vi "Taiko_Init.vi"(8 "error in (no error)":errorcluster, 9 "LBLHFeaturesRef":refnum<vi>, 10 "LBSysStatRef":refnum<vi>, 11 "Data":T1 {"TaggedValueList"."Tag" format="%x" items=["NONE"=0, "Locked"=16, "SoftLock"=17, "KeyLock"=18, "Class_IV_Lock"=20, "Interlock"=24, "LaserMode"=32, "LDH_PulsePowerTable"=33, "TriggerMode"=48, "TriggerLevelRaw"=64, "TriggerLevelRawLoLimit"=65, "TriggerLevelRawHiLimit"=66, "TriggerLevel"=72, "TriggerLevelLoLimit"=73, "TriggerLevelHiLimit"=74, "FastGate"=80, "FastGateImp"=96, "SlowGate"=112, "TargetTempRaw"=144, "TargetTempRawLoLimit"=145, "TargetTempRawHiLimit"=146, "CurrentTempRaw"=148, "CaseTempRaw"=149, "TargetTemp"=152, "TargetTempLoLimit"=153, "TargetTempHiLimit"=154, "CurrentTemp"=156, "CaseTemp"=157, "TempScale"=159, "Frequency"=168, "FrequencyLoLimit"=169, "FrequencyHiLimit"=170, "PulsePowerRaw"=176, "PulsePowerRawLoLimit"=177, "PulsePowerRawHiLimit"=178, "PulsePowerPermille"=180, "PulseShape"=181, "PulsePower"=184, "PulsePowerLoLimit"=185, "PulsePowerHiLimit"=186, "PulsePowerNanowatt"=188, "PulsePowerVoltage"=190, "PulseEnergy"=191, "CwPowerRaw"=192, "CwPowerRawLoLimit"=193, "CwPowerRawHiLimit"=194, "CwPowerPermille"=196, "CwPower"=200, "CwPowerLoLimit"=201, "CwPowerHiLimit"=202, "CwPowerMicroWatt"=204, "BurstLen"=208, "BurstPeriod"=224, "LDH_Fan"=240, "UI_Exclusive"=256]}) -> (0 "error out":errorcluster, 1 "Status":string, 2 "LHInfoData":string[][](array[string]), 3 "Data out":T1 {"TaggedValueList"."Tag" format="%x" items=["NONE"=0, "Locked"=16, "SoftLock"=17, "KeyLock"=18, "Class_IV_Lock"=20, "Interlock"=24, "LaserMode"=32, "LDH_PulsePowerTable"=33, "TriggerMode"=48, "TriggerLevelRaw"=64, "TriggerLevelRawLoLimit"=65, "TriggerLevelRawHiLimit"=66, "TriggerLevel"=72, "TriggerLevelLoLimit"=73, "TriggerLevelHiLimit"=74, "FastGate"=80, "FastGateImp"=96, "SlowGate"=112, "TargetTempRaw"=144, "TargetTempRawLoLimit"=145, "TargetTempRawHiLimit"=146, "CurrentTempRaw"=148, "CaseTempRaw"=149, "TargetTemp"=152, "TargetTempLoLimit"=153, "TargetTempHiLimit"=154, "CurrentTemp"=156, "CaseTemp"=157, "TempScale"=159, "Frequency"=168, "FrequencyLoLimit"=169, "FrequencyHiLimit"=170, "PulsePowerRaw"=176, "PulsePowerRawLoLimit"=177, "PulsePowerRawHiLimit"=178, "PulsePowerPermille"=180, "PulseShape"=181, "PulsePower"=184, "PulsePowerLoLimit"=185, "PulsePowerHiLimit"=186, "PulsePowerNanowatt"=188, "PulsePowerVoltage"=190, "PulseEnergy"=191, "CwPowerRaw"=192, "CwPowerRawLoLimit"=193, "CwPowerRawHiLimit"=194, "CwPowerPermille"=196, "CwPower"=200, "CwPowerLoLimit"=201, "CwPowerHiLimit"=202, "CwPowerMicroWatt"=204, "BurstLen"=208, "BurstPeriod"=224, "LDH_Fan"=240, "UI_Exclusive"=256]}, 4 "Features":string)   [LabVIEW 2017]
uses:
  Types/Taiko_Data.ctl
  _lib/PDLM/pdlm_lib_x86_x64_UIThread.llb/PDLM_TaggedValueList.ctl
  _lib/PDLM/pdlm_lib_x86_x64_UIThread.llb/PDLM_TaggedValue.ctl
  _lib/PDLM/pdlm_lib_x86_x64_UIThread.llb/PDLM_Tag.ctl
  Types/ControlAttributes.ctl
  Types/ScaleDisplayParams.ctl
  _lib/PDLM/pdlm_lib_x86_x64_UIThread.llb/PDLM_LHFeatures.ctl
  _lib/PDLM/pdlm_lib_x86_x64_UIThread.llb/PDLM_NamedBit.ctl
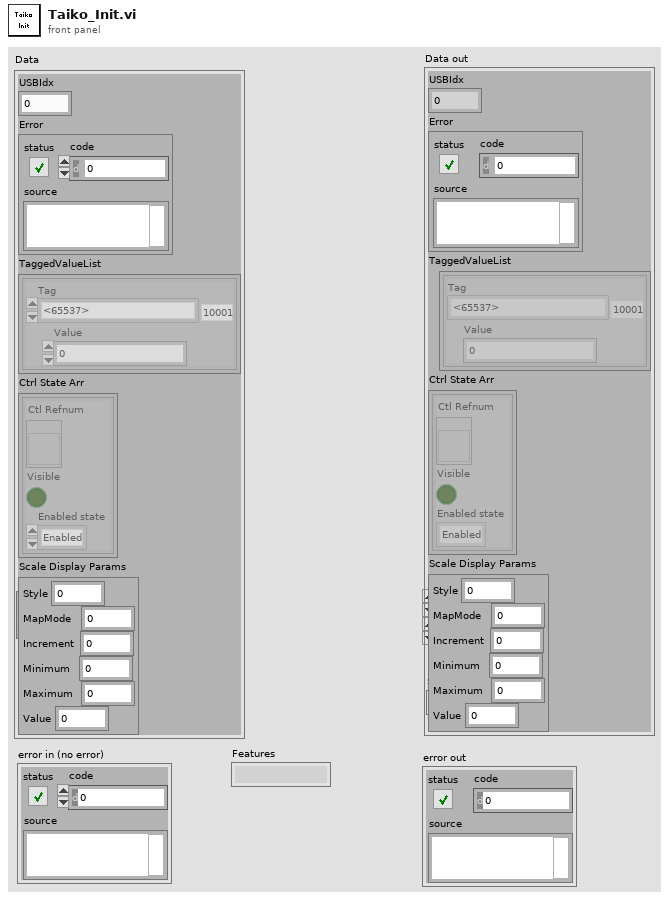
[diagram p1: front panel]
types:
  T1 = typedef "Taiko_Data.ctl" = cluster{"USBIdx":i32, "Error":errorcluster, "TaggedValueList":T2, "Ctrl State Arr":T5[], "Scale Display Params":T6}
  T2 = typedef "PDLM_TaggedValueList.ctl" = T3[]
  T3 = typedef "PDLM_TaggedValue.ctl" = cluster{"Tag":T4, "Value":u32}
  T4 = typedef "PDLM_Tag.ctl" = u32
  T5 = typedef "ControlAttributes.ctl" = cluster{"Ctl Refnum":refnum<vi>, "Visible":bool, "Enabled state":enum8{"Enabled", "Disabled", "Disabled and Grayed Out"}}
  T6 = typedef "ScaleDisplayParams.ctl" = cluster{"Style":u8, "MapMode":u8, "Increment":dbl, "Minimum":dbl, "Maximum":dbl, "Value":dbl}
  T7 = typedef "PDLM_LHFeatures.ctl" = T8[]
  T8 = typedef "PDLM_NamedBit.ctl" = cluster{"StatName":string, "StatBit":bool}
  T9 = typedef "LVStringsAndValuesArrayTypeDef_U32.ctl" = cluster{"String":string, "Value":u32}[]
  T10 = typedef "PDLM_LHInfo.ctl" = cluster{"LType":string, "Date":string, "LClass":string}
  T11 = typedef "PDLM_LHData.ctl" = cluster{"SerNo":u32, "Features":u32, "FreqMin":u32, "FreqMax":u32, "CwPowerMax":u32, "PulsePowerMax":u32, "WavelengthNominal":u16, "CaseTempMax":u16, "Protection":bool, "LHTypeCtrlVoltage":u16, "LHMaxVoltage":u16, "CurrentTEP12V":u16, "LaserType":T12, "LHVersion":T13, "CalWarrentHours":u16}
  T12 = typedef "PDLM_LHData_LaserType.ctl" = u16
  T13 = typedef "PDLM_LHVersion.ctl" = cluster{"Major":u16, "Minor":u16}
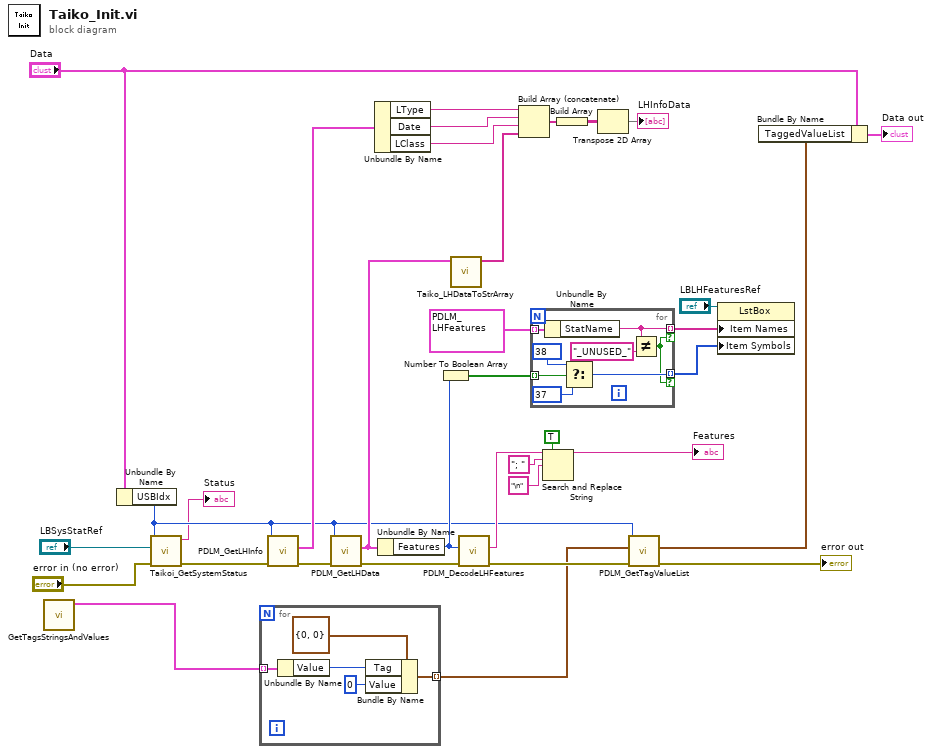
[diagram p0: block diagram]
diagram:
  n1 = call "GetTagsStringsAndValues.vi"() -> ("Strings And Values []"=w1:T9)  [unwired: 11 in]
  n2 = Unbundle By Name("Data") -> ("USBIdx"=w6:i32)
  n3 = call "Taikoi_GetSystemStatus.vi"("error in (no error)"="error in (no error)", "LBSysStatRef"="LBSysStatRef", "USBIdx"=w6) -> ("error out"=w7:errorcluster, "Status"=→"Status":string)  [unwired: 5 in, 2 out]
  n4 = for {
    tunnel: w1 -> [w39] mode=indexing
    tunnel: [w35] -> w11 mode=indexing
    n5 = Unbundle By Name(w39) -> ("Value"=w37:u32)
    n6 = Bundle By Name(cluster=T3 {"Tag"=0, "Value"=0} ("TaggedValue"), "Tag"=w37, "Value"=u32 0) -> (w35:T3)
  }
  n7 = call "PDLM_GetLHInfo.vi"("error in (no error)"=w7, "USBIdx"=w6) -> ("error out"=w34:errorcluster, "LHInfo"=w29:T10)  [unwired: 7 in, 1 out]
  n8 = call "PDLM_GetLHData.vi"("error in (no error)"=w34, "USBIdx"=w6) -> ("error out"=w27:errorcluster, "Data"=w28:T11)  [unwired: 7 in, 1 out]
  n9 = Unbundle By Name(w29) -> ("LType"=w4:string, "Date"=w3:string, "LClass"=w2:string)
  n10 = Unbundle By Name(w28) -> ("Features"=w23:u32)
  n11 = Number To Boolean Array(number=w23) -> (Boolean array=w24:bool[])
  n12 = call "Taiko_LHDataToStrArray.vi"("LHData"=w28) -> ("StrArray"=w32:string[])  [unwired: 10 in]
  n13 = call "PDLM_DecodeLHFeatures.vi"("error in (no error)"=w27, "features"=w23) -> ("error out"=w26:errorcluster, "Buffer"=w15:string)  [unwired: 7 in, 1 out]
  n14 = Build Array (concatenate)(w4, w3, w2, w32) -> (w30:string[])
  n15 = for {
    tunnel: w24 -> [w46] mode=indexing
    tunnel: T7 [{"StatName"="CW_CAPABILITY", "StatBit"=FALSE}, {"StatName"="_UNUSED_", "StatBit"=FALSE}, {"StatName"="_UNUSED_", "StatBit"=FALSE}, {"StatName"="_UNUSED_", "StatBit"=FALSE}, {"StatName"="BURST_CAPABILITY", "StatBit"=FALSE}, {"StatName"="_UNUSED_", "StatBit"=FALSE}, {"StatName"="EXTERNAL_TRIGGERABLE_BURSTS", "StatBit"=FALSE}, {"StatName"="EXTERNAL_TRIGGERABLE_PULSES", "StatBit"=FALSE}, {"StatName"="WL_TUNABLE", "StatBit"=FALSE}, {"StatName"="_UNUSED_", "StatBit"=FALSE}, {"StatName"="_UNUSED_", "StatBit"=FALSE}, {"StatName"="_UNUSED_", "StatBit"=FALSE}, {"StatName"="_UNUSED_", "StatBit"=FALSE}, {"StatName"="_UNUSED_", "StatBit"=FALSE}, {"StatName"="_UNUSED_", "StatBit"=FALSE}, {"StatName"="_UNUSED_", "StatBit"=FALSE}, {"StatName"="COOLING_FAN", "StatBit"=FALSE}, {"StatName"="SWITCHABLE_FAN", "StatBit"=FALSE}, {"StatName"="_UNUSED_", "StatBit"=FALSE}, {"StatName"="_UNUSED_", "StatBit"=FALSE}, {"StatName"="_UNUSED_", "StatBit"=FALSE}, {"StatName"="_UNUSED_", "StatBit"=FALSE}, {"StatName"="_UNUSED_", "StatBit"=FALSE}, {"StatName"="_UNUSED_", "StatBit"=FALSE}, {"StatName"="_UNUSED_", "StatBit"=FALSE}, {"StatName"="_UNUSED_", "StatBit"=FALSE}, {"StatName"="_UNUSED_", "StatBit"=FALSE}, {"StatName"="_UNUSED_", "StatBit"=FALSE}, {"StatName"="_UNUSED_", "StatBit"=FALSE}, {"StatName"="_UNUSED_", "StatBit"=FALSE}, {"StatName"="_UNUSED_", "StatBit"=FALSE}, {"StatName"="_UNUSED_", "StatBit"=FALSE}] ("LHFeatures") -> [w47] mode=indexing
    tunnel: [w42] -> w21 mode=indexing if=w40
    tunnel: [w43] -> w20 mode=indexing if=w40
    n16 = Unbundle By Name(w47) -> ("StatName"=w42:string)
    n17 = Select(t=38, s=w46, f=37) -> (s? t:f=w43:i32)
    n18 = Not Equal?(x=w42, y="_UNUSED_") -> (x != y?=w40:bool)
  }
  n19 = Search and Replace String(replace all?=TRUE ("replace all? (F)"), input string=w15, search string="; ", replace string="\n" ("replace string (\"\")")) -> (result string=→"Features":string)  [unwired: 4 in, 3 out]
  n20 = Build Array(w30) -> (w31:string[][])
  n21 = Transpose 2D Array(2D array=w31) -> (transposed array=→"LHInfoData":string[][])
  n22 = call "PDLM_GetTagValueList.vi"("error in (no error)"=w26, "TaggedValueList"=w11, "USBIdx"=w6) -> ("error out"=→"error out":errorcluster, "TaggedValueList out"=w12:T2)  [unwired: 6 in, 1 out]
  n23 = property class="LstBox"(reference="LBLHFeaturesRef", "Item Names"=w21, "Item Symbols"=w20) -> ()  [unwired: 1 in, 2 out]
  n24 = Bundle By Name(cluster="Data", "TaggedValueList"=w12) -> (→"Data out":T1)
